vi "Simulator.vi"(0 "Simulator Data Out":T1(array[cluster]), 3 "Sample Size":cluster{"Width (µm)":dbl, "Height (µm)":dbl}={"Width (µm)"=40.0, "Height (µm)"=40.0}, 4 "error in (no error)":errorcluster, 5 "Distance Between Interpolated Points":dbl) -> (1 "error out":errorcluster)   [LabVIEW 2013]
doc: "This VI controls the simulator."
uses:
  Global Variables.vi
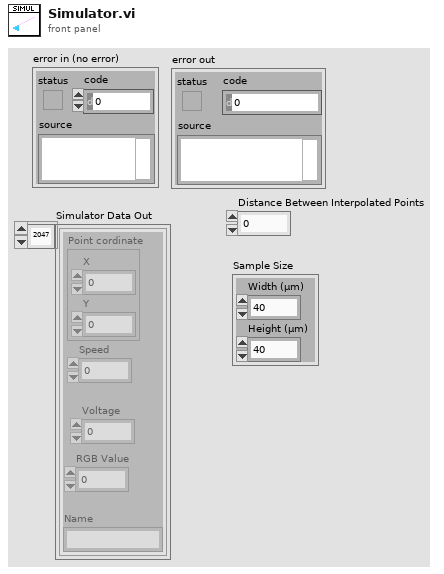
[diagram p1: front panel]
types:
  T1 = cluster{"Point cordinate":cluster{"X":dbl, "Y":dbl}, "Speed":dbl, "Voltage":dbl, "RGB Value":i32, "Name":string}[]
  T2 = cluster{"Point cordinate":cluster{"X":dbl, "Y":dbl}, "Speed":dbl, "Voltage":dbl, "RGB Value":i32, "Name":string}
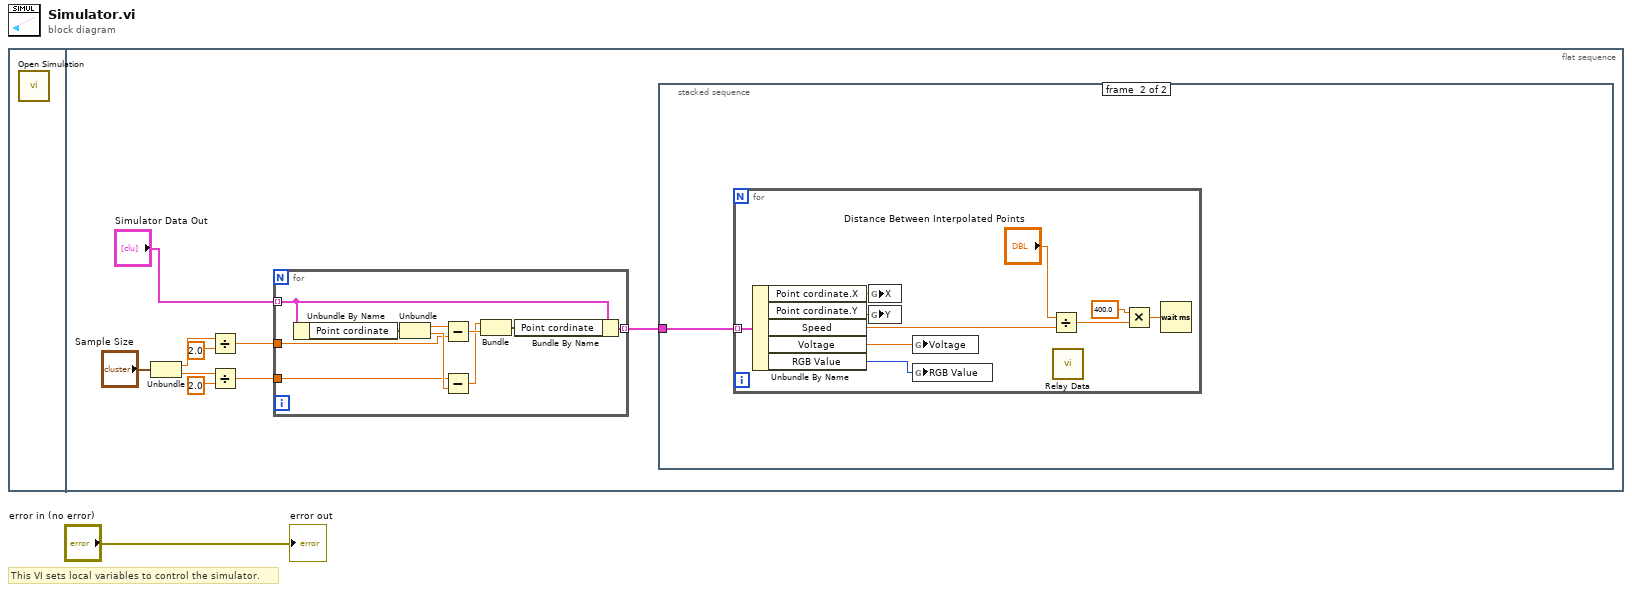
[diagram p0: block diagram]
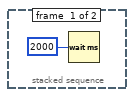
[diagram p2: hidden frame]
diagram:
  # "This VI sets local variables to control the simulator."
  n1 = flat-sequence {
    frame #0 {
      n2 = call "Open Simulation.vi"() -> ()  [unwired: 12 in]
    }
    frame #1 {
      n3 = Unbundle("Sample Size") -> ("Width (µm)"=w10:dbl, "Height (µm)"=w5:dbl)
      n4 = Divide(x=w10, y=2.0) -> (x/y=w7:dbl)
      n5 = Divide(x=w5, y=2.0) -> (x/y=w4:dbl)
      n6 = for {
        tunnel: "Simulator Data Out" -> [w11] mode=indexing
        tunnel: [w18] -> w3 mode=indexing
        tunnel: w7 -> [w13]
        tunnel: w4 -> [w12]
        n7 = Unbundle By Name(w11) -> ("Point cordinate"=w20:cluster{"X":dbl, "Y":dbl})
        n8 = Unbundle(w20) -> ("X"=w17:dbl, "Y"=w14:dbl)
        n9 = Subtract(x=w17, y=w13) -> (x-y=w16:dbl)
        n10 = Subtract(x=w12, y=w14) -> (x-y=w15:dbl)
        n11 = Bundle(w15, w16) -> (w19:cluster{dbl, dbl})  [unwired: 1 in]
        n12 = Bundle By Name(cluster=w11, "Point cordinate"=w19) -> (w18:T2)
      }
      n13 = stacked-sequence {
        tunnel: w3 -> [_ w22]
        frame #0 {
          n14 = Wait (ms)(milliseconds to wait=u32 2000) -> ()  [unwired: 1 out]
        }
        frame #1 {
          n15 = for {
            tunnel: w22 -> [w30] mode=indexing
            n16 = Unbundle By Name(w30) -> ("Point cordinate.X"=w31:dbl, "Point cordinate.Y"=w32:dbl, "Speed"=w29:dbl, "Voltage"=w28:dbl, "RGB Value"=w27:i32)
            n17 = global write "Global Variables.vi" "X"(w31) -> ()
            n18 = global write "Global Variables.vi" "Y"(w32) -> ()
            n19 = global write "Global Variables.vi" "Voltage"(w28) -> ()
            n20 = global write "Global Variables.vi" "RGB Value"(w27) -> ()
            n21 = Divide(x="Distance Between Interpolated Points", y=w29) -> (x/y=w26:dbl)
            n22 = call "Relay Data.vi"() -> ()  [unwired: 12 in]
            n23 = Multiply(x=400.0, y=w26) -> (x*y=w24:dbl)
            n24 = Wait (ms)(milliseconds to wait=w24) -> ()  [unwired: 1 out]
          }
        }
      }
    }
  }
  "error out" <- "error in (no error)"
